vi "Data Access Client_1.vi"() -> ()   [LabVIEW 2019]
uses:
  subVIs/Az-Ctrl.ctl
  subVIs/Alt-Ctrl.ctl
  subVIs/HSB-Ctrl.ctl
  subVIs/Fork Panel-Ctrl.ctl
  subVIs/UPS-Ctrl.ctl
  subVIs/Alarm-Ctrl.ctl
  <vilib>/OPCUA/NI OPC UA Client.lvlib
panel:
  out "Alarm Warnings":T7
  out "Alarm Errors":T8
  in  "stop":bool
  in  "security policy":T9
  in  "server endpoint URL":string="opc.tcp://INOCS:55101"
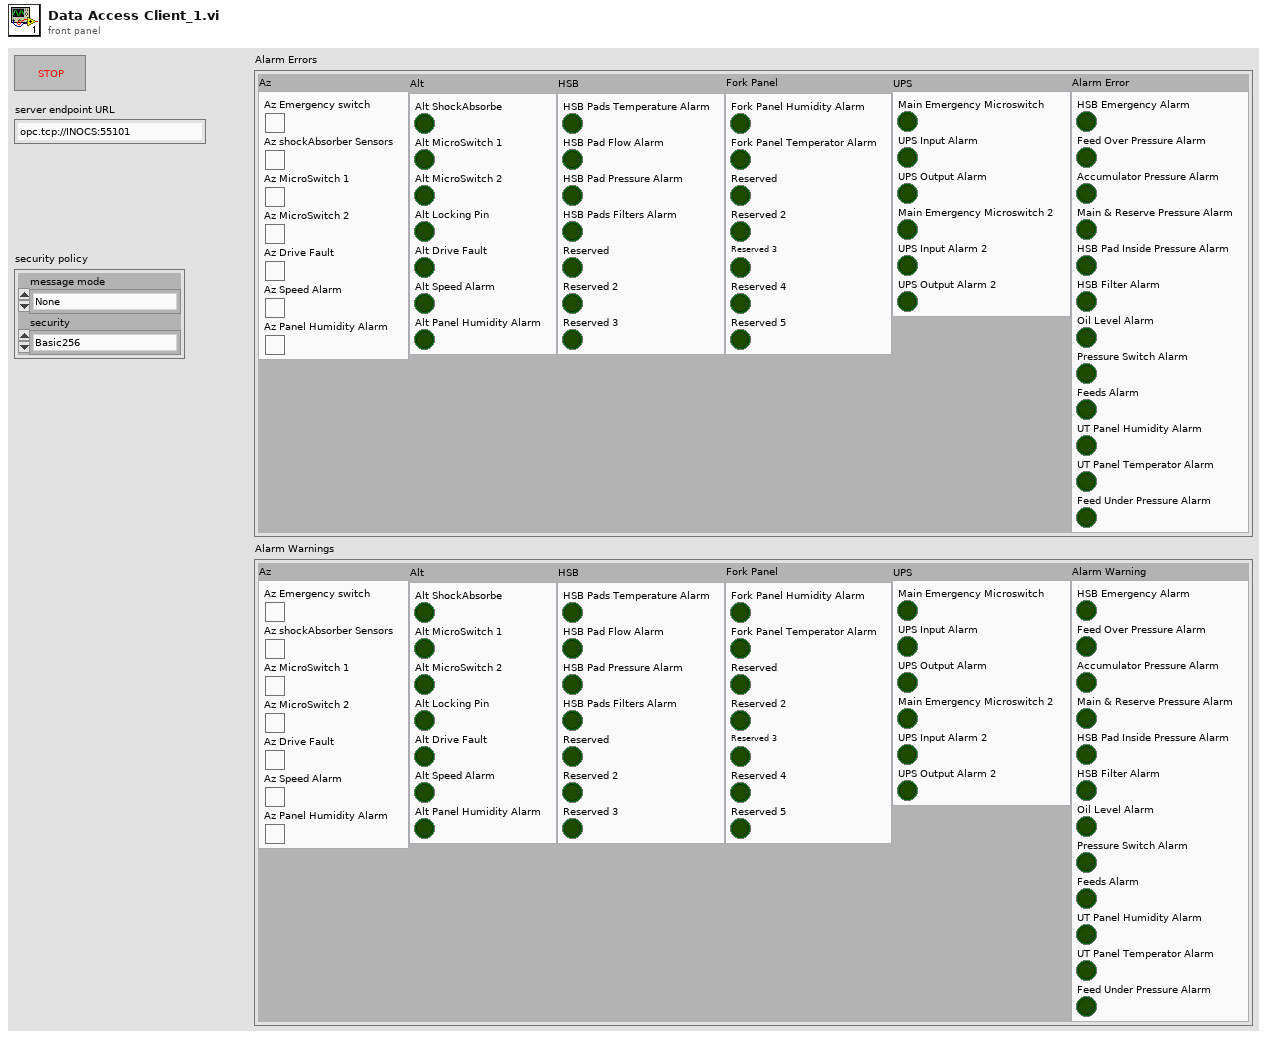
[diagram p1: front panel]
types:
  T1 = typedef "Az-Ctrl.ctl" = cluster{"Az Emergency switch":bool, "Az shockAbsorber Sensors":bool, "Az MicroSwitch 1":bool, "Az MicroSwitch 2":bool, "Az Drive Fault":bool, "Az Speed Alarm":bool, "Az Panel Humidity Alarm":bool}
  T2 = typedef "Alt-Ctrl.ctl" = cluster{"Alt ShockAbsorbe":bool, "Alt MicroSwitch 1":bool, "Alt MicroSwitch 2":bool, "Alt Locking Pin":bool, "Alt Drive Fault":bool, "Alt Speed Alarm":bool, "Alt Panel Humidity Alarm":bool}
  T3 = typedef "HSB-Ctrl.ctl" = cluster{"HSB Pads Temperature Alarm":bool, "HSB Pad Flow Alarm":bool, "HSB Pad Pressure Alarm":bool, "HSB Pads Filters Alarm":bool, "Reserved":bool, "Reserved 2":bool, "Reserved 3":bool}
  T4 = typedef "Fork Panel-Ctrl.ctl" = cluster{"Fork Panel Humidity Alarm":bool, "Fork Panel Temperator Alarm":bool, "Reserved":bool, "Reserved 2":bool, "Reserved 3":bool, "Reserved 4":bool, "Reserved 5":bool}
  T5 = typedef "UPS-Ctrl.ctl" = cluster{"Main Emergency Microswitch":bool, "UPS Input Alarm":bool, "UPS Output Alarm":bool, "Main Emergency Microswitch 2":bool, "UPS Input Alarm 2":bool, "UPS Output Alarm 2":bool}
  T6 = typedef "Alarm-Ctrl.ctl" = cluster{"HSB Emergency Alarm":bool, "Feed Over Pressure Alarm":bool, "Accumulator Pressure Alarm":bool, "Main & Reserve Pressure Alarm":bool, "HSB Pad Inside Pressure Alarm":bool, "HSB Filter Alarm":bool, "Oil Level Alarm":bool, "Pressure Switch Alarm":bool, "Feeds Alarm":bool, "UT Panel Humidity Alarm":bool, "UT Panel Temperator Alarm":bool, "Feed Under Pressure Alarm":bool}
  T7 = cluster{"Az":T1, "Alt":T2, "HSB":T3, "Fork Panel":T4, "UPS":T5, "Alarm Warning":T6}
  T8 = cluster{"Az":T1, "Alt":T2, "HSB":T3, "Fork Panel ":T4, "UPS":T5, "Alarm Error":T6}
  T9 = cluster{"message mode":enum16{"None", "Sign", "Sign and Encrypt"}, "security":enum16{"Basic256", "Basic128Rsa15"}}
  T10 = typedef "OPC UA Client Refnum.ctl" = refnum<k21>
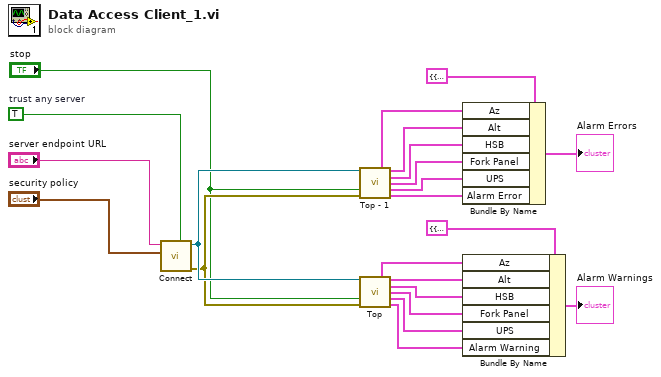
[diagram p0: block diagram]
diagram:
  w20 = TRUE  # trust any server
  n1 = call <vilib>:"Connect.vi"("trust any server (F)"=w20, "security policy"="security policy", "server endpoint URL"="server endpoint URL") -> ("error out"=w18:errorcluster, "OPC UA client refnum out"=w19:T10)  [unwired: 6 in, 1 out]
  n2 = call "Top - 1.vi"("OPC UA client refnum out"=w19, "stop"="stop", "error IO"=w18) -> ("Az"=w16:T1, "Alt"=w15:T2, "HSB"=w14:T3, "Fork Panel"=w13:T4, "UPS"=w12:T5, "Alarm Warning"=w11:T6)  [unwired: 7 in]
  n3 = call "Top.vi"("OPC UA client refnum out"=w19, "stop"="stop", "error IO"=w18) -> ("Az"=w8:T1, "Alt"=w7:T2, "HSB"=w6:T3, "Fork Panel"=w5:T4, "UPS"=w4:T5, "Alarm Error"=w3:T6)  [unwired: 7 in]
  n4 = Bundle By Name(cluster=T8 {"Az"={"Az Emergency switch"=FALSE, "Az shockAbsorber Sensors"=FALSE, "Az MicroSwitch 1"=FALSE, "Az MicroSwitch 2"=FALSE, "Az Drive Fault"=FALSE, "Az Speed Alarm"=FALSE, "Az Panel Humidity Alarm"=FALSE}, "Alt"={"Alt ShockAbsorbe"=FALSE, "Alt MicroSwitch 1"=FALSE, "Alt MicroSwitch 2"=FALSE, "Alt Locking Pin"=FALSE, "Alt Drive Fault"=FALSE, "Alt Speed Alarm"=FALSE, "Alt Panel Humidity Alarm"=FALSE}, "HSB"={"HSB Pads Temperature Alarm"=FALSE, "HSB Pad Flow Alarm"=FALSE, "HSB Pad Pressure Alarm"=FALSE, "HSB Pads Filters Alarm"=FALSE, "Reserved"=FALSE, "Reserved 2"=FALSE, "Reserved 3"=FALSE}, "Fork Panel "={"Fork Panel Humidity Alarm"=FALSE, "Fork Panel Temperator Alarm"=FALSE, "Reserved"=FALSE, "Reserved 2"=FALSE, "Reserved 3"=FALSE, "Reserved 4"=FALSE, "Reserved 5"=FALSE}, "UPS"={"Main Emergency Microswitch"=FALSE, "UPS Input Alarm"=FALSE, "UPS Output Alarm"=FALSE, "Main Emergency Microswitch 2"=FALSE, "UPS Input Alarm 2"=FALSE, "UPS Output Alarm 2"=FALSE}, "Alarm Error"={"HSB Emergency Alarm"=FALSE, "Feed Over Pressure Alarm"=FALSE, "Accumulator Pressure Alarm"=FALSE, "Main & Reserve Pressure Alarm"=FALSE, "HSB Pad Inside Pressure Alarm"=FALSE, "HSB Filter Alarm"=FALSE, "Oil Level Alarm"=FALSE, "Pressure Switch Alarm"=FALSE, "Feeds Alarm"=FALSE, "UT Panel Humidity Alarm"=FALSE, "UT Panel Temperator Alarm"=FALSE, "Feed Under Pressure Alarm"=FALSE}} ("Alarm Errors"), "Az"=w16, "Alt"=w15, "HSB"=w14, "Fork Panel"=w13, "UPS"=w12, "Alarm Error"=w11) -> (→"Alarm Errors":T8)
  n5 = Bundle By Name(cluster=T7 {"Az"={"Az Emergency switch"=FALSE, "Az shockAbsorber Sensors"=FALSE, "Az MicroSwitch 1"=FALSE, "Az MicroSwitch 2"=FALSE, "Az Drive Fault"=FALSE, "Az Speed Alarm"=FALSE, "Az Panel Humidity Alarm"=FALSE}, "Alt"={"Alt ShockAbsorbe"=FALSE, "Alt MicroSwitch 1"=FALSE, "Alt MicroSwitch 2"=FALSE, "Alt Locking Pin"=FALSE, "Alt Drive Fault"=FALSE, "Alt Speed Alarm"=FALSE, "Alt Panel Humidity Alarm"=FALSE}, "HSB"={"HSB Pads Temperature Alarm"=FALSE, "HSB Pad Flow Alarm"=FALSE, "HSB Pad Pressure Alarm"=FALSE, "HSB Pads Filters Alarm"=FALSE, "Reserved"=FALSE, "Reserved 2"=FALSE, "Reserved 3"=FALSE}, "Fork Panel"={"Fork Panel Humidity Alarm"=FALSE, "Fork Panel Temperator Alarm"=FALSE, "Reserved"=FALSE, "Reserved 2"=FALSE, "Reserved 3"=FALSE, "Reserved 4"=FALSE, "Reserved 5"=FALSE}, "UPS"={"Main Emergency Microswitch"=FALSE, "UPS Input Alarm"=FALSE, "UPS Output Alarm"=FALSE, "Main Emergency Microswitch 2"=FALSE, "UPS Input Alarm 2"=FALSE, "UPS Output Alarm 2"=FALSE}, "Alarm Warning"={"HSB Emergency Alarm"=FALSE, "Feed Over Pressure Alarm"=FALSE, "Accumulator Pressure Alarm"=FALSE, "Main & Reserve Pressure Alarm"=FALSE, "HSB Pad Inside Pressure Alarm"=FALSE, "HSB Filter Alarm"=FALSE, "Oil Level Alarm"=FALSE, "Pressure Switch Alarm"=FALSE, "Feeds Alarm"=FALSE, "UT Panel Humidity Alarm"=FALSE, "UT Panel Temperator Alarm"=FALSE, "Feed Under Pressure Alarm"=FALSE}} ("Alarm Warnings"), "Az"=w8, "Alt"=w7, "HSB"=w6, "Fork Panel"=w5, "UPS"=w4, "Alarm Warning"=w3) -> (→"Alarm Warnings":T7)
